vi "lv os independant username.vi"(8 "error in (no error)":errorcluster) -> (0 "error out":errorcluster, 2 "Application:User Name":string)   [LabVIEW 2022 SP3]
panel:
  # "this only works when the labview preferences History have the login name enabled"
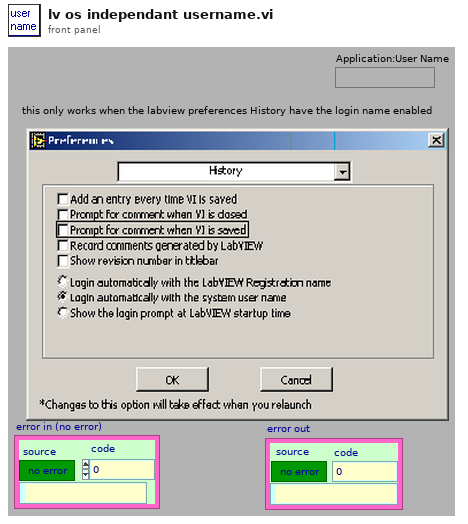
[diagram p1: front panel]
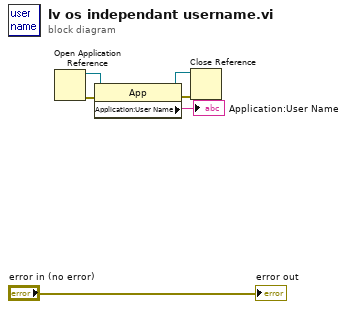
[diagram p0: block diagram]
diagram:
  n1 = Open Application Reference() -> (0:w5:errorcluster, 3:w6:refnum<vi>)  [unwired: 4 in]
  n2 = property class="App"(reference=w6, error in=w5) -> (reference out=w4:refnum<vi>, error out=w3:errorcluster, "Application:User Name"=→"Application:User Name":string)
  n3 = Close Reference(reference=w4, error in (no error)=w3) -> ()  [unwired: 1 out]
  "error out" <- "error in (no error)"
